vi "Cutlogfiles.vi"() -> ()   [LabVIEW 2018]
uses:
  <vilib>/Enthought/Python Integration Toolkit/api/Console Visibility.ctl
  Global Variables.vi
  <vilib>/Enthought/Python Integration Toolkit/Python Integration Toolkit.lvlib
panel:
  in  "Sample Rate":i32=100
  in  "New file":bool
  in  "selected path":path=path "C:/Labview Test Data/2018-08-13/Sensors/Log_Sensors_DAQ_0.tdms"
  out "XY Graph 2":cluster{dbl, "YScale.Maximum":dbl}[](graph)=[{3617058104.92992, "YScale.Maximum"=0.02}, {3617058117.2644606, "YScale.Maximum"=0.02}]
  out "XY Graph":cluster{dbl[], dbl[]}(graph)={[3617058104.92992, 3617058105.071405, 3617058105.204719, 3617058105.339352, 3617058105.4654217, 3617058105.5895977, 3617058105.723924, 3617058105.8577886, 3617058105.9931545, 3617058106.126216, 3617058106.2686815, 3617058106.402235, 3617058106.5402184, 3617058106.6768394, 3617058106.8146977, 3617058106.9502025, 3617058107.086078, 3617058107.2211895, 3617058107.3549776, 3617058107.4918585, 3617058107.627911, 3617058107.762443, 3617058107.901148, 3617058108.034609, 3617058108.171561, 3617058108.3105903, 3617058108.448009, 3617058108.586817, 3617058108.725321, 3617058108.86412, 3617058108.9984703, 3617058109.136935, 3617058109.275936, 3617058109.415624, 3617058109.5444145, 3617058109.6839633, 3617058109.8212304, 3617058109.959656, 3617058110.099505, 3617058110.2352777, 3617058110.37625, 3617058110.5166783, 3617058110.654278, 3617058110.792069, 3617058110.9294696, 3617058111.0667214, 3617058111.2080984, 3617058111.3436384, 3617058111.4812026, 3617058111.6171255, 3617058111.754656, 3617058111.8906007, 3617058112.028036, 3617058112.1654263, 3617058112.3010263, 3617058112.437075, 3617058112.5742207, 3617058112.7098174, 3617058112.847483, 3617058112.984029, 3617058113.11964, 3617058113.256136, 3617058113.395491, 3617058113.5323257, 3617058113.6705136, 3617058113.8095255, 3617058113.945854, 3617058114.0845695, 3617058114.2227335, 3617058114.360228, 3617058114.496631, 3617058114.634196, 3617058114.77004, 3617058114.90852, 3617058115.0450034, 3617058115.1819854, 3617058115.318167, 3617058115.4536457, 3617058115.591485, 3617058115.7283754, 3617058115.870709, 3617058116.009808, 3617058116.147975, 3617058116.2889624, 3617058116.4316134, 3617058116.575004, 3617058116.7180977, 3617058116.860796, 3617058117.000852, 3617058117.1353416, 3617058117.2644606], array[9200 elements]}
  out "Selected Channel":u32=2
  in  "stop":bool
  in  "Array":string[](array[string])=["Current_0", "Current_1", "Current_2", "Current_3", "Current_4", "Current_5", "Current_6", "Current_7"]
  in  "Cut":bool
  in  "Final Time":timestamp=timestamp(3617058117.2644606 s since 1904-01-01) format="%<%X\n%x>T"
  in  "Inital Time":timestamp=timestamp(3617058104.92992 s since 1904-01-01) format="%<%X\n%x>T"
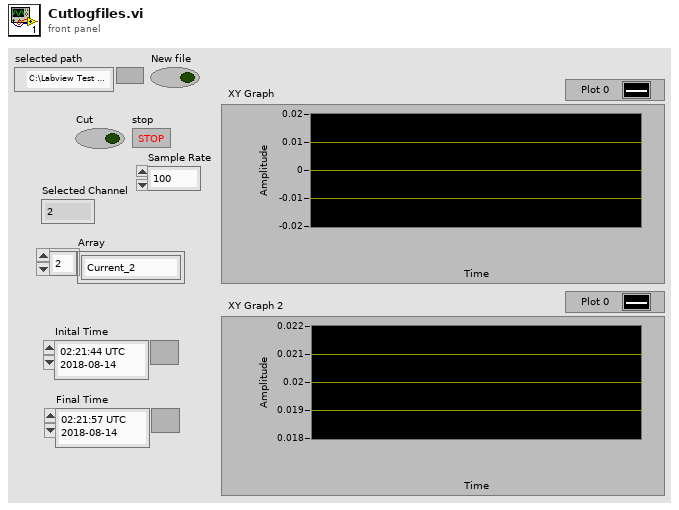
[diagram p1: front panel]
types:
  T1 = typedef "Python Integration Toolkit.lvlib/Console Visibility.ctl" = enum16{"Show Console", "Show Console While Running", "Hide Console"}
  T2 = enum16{"open", "open or create", "create or replace", "create", "open (read-only)"}
  T3 = typedef "Python Integration Toolkit.lvlib/Session ID.ctl" = u64
  T4 = typedef "Python Integration Toolkit.lvlib/Python Objects.ctl" = variant
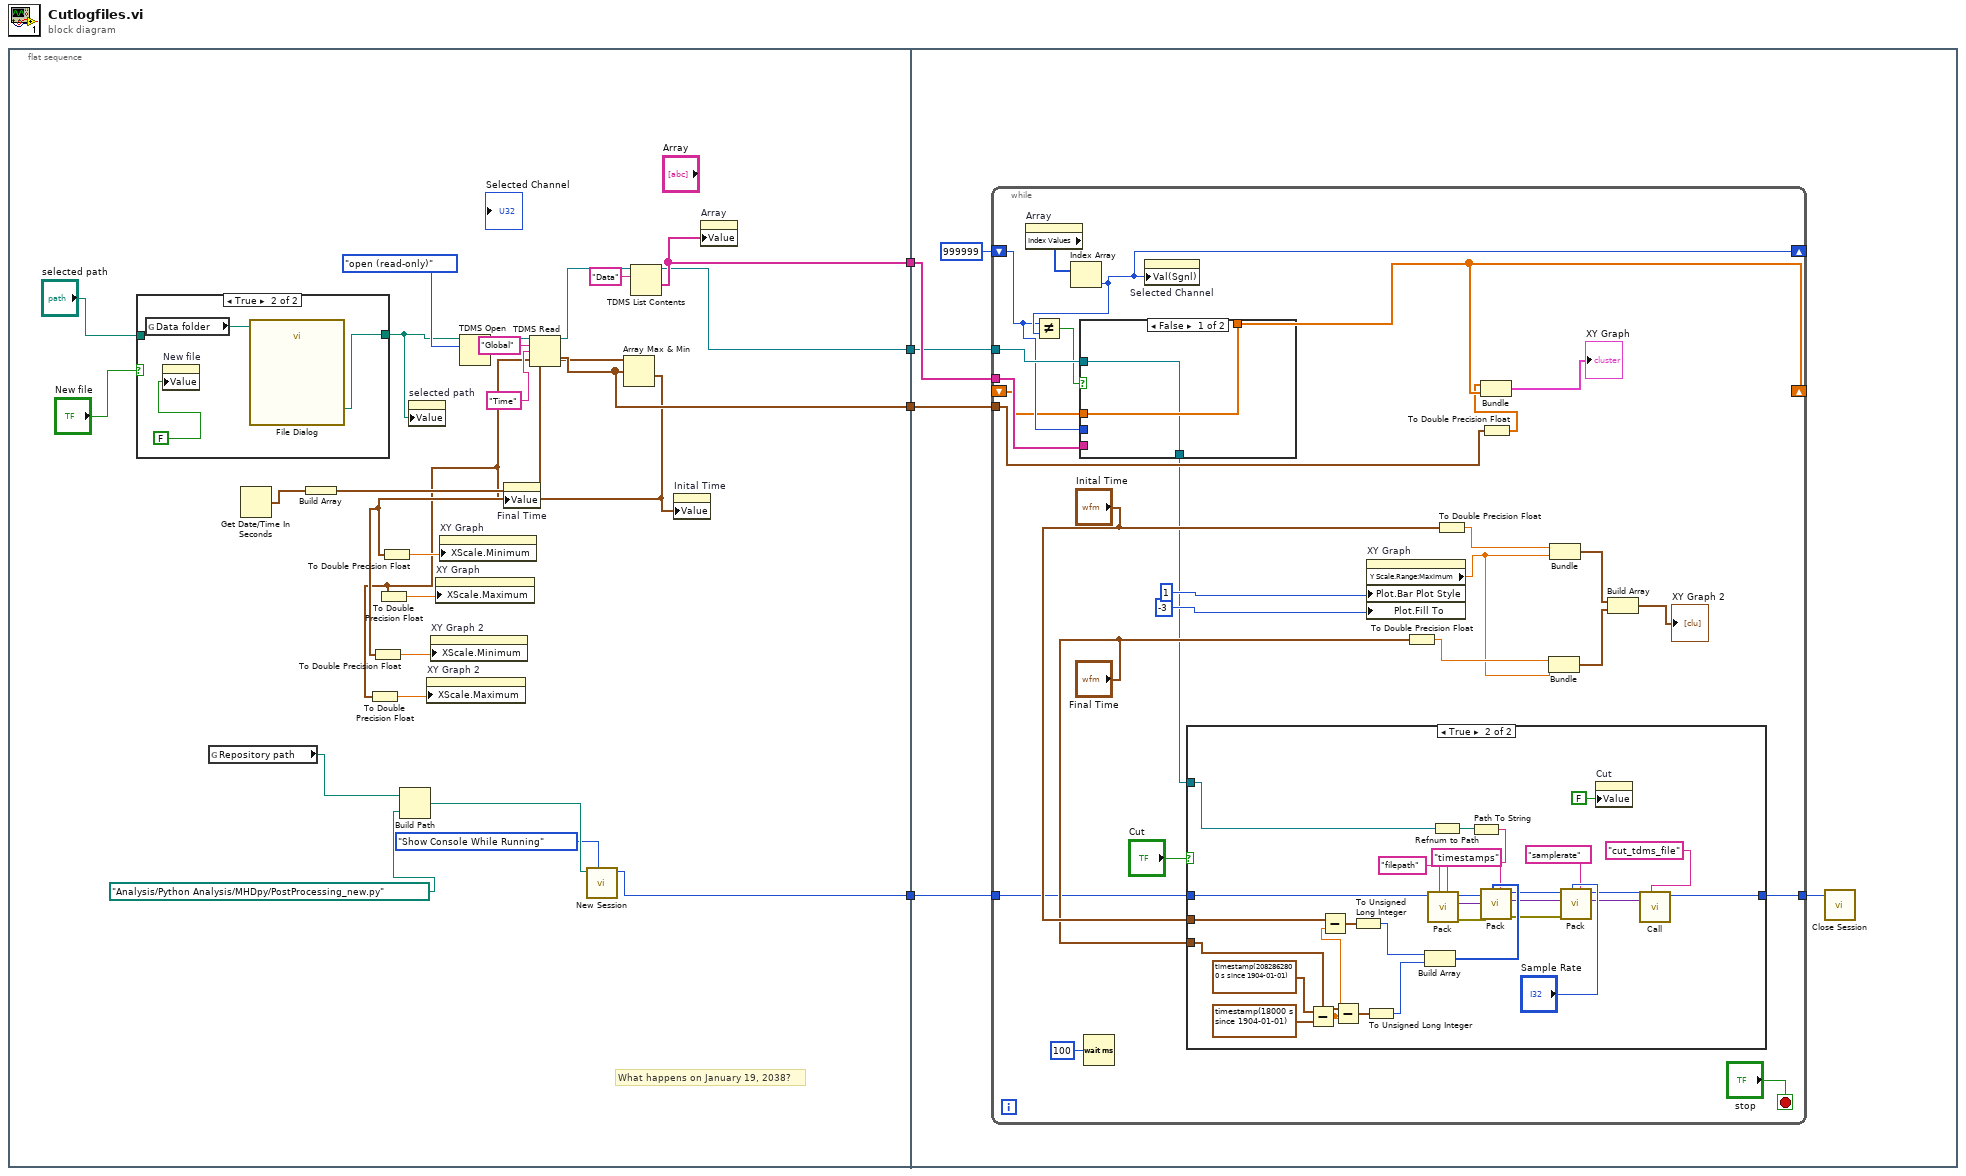
[diagram p0: block diagram]
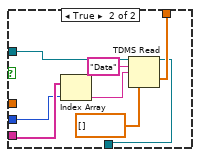
[diagram p4: hidden frame]
diagram:
  n1 = flat-sequence {
    tunnel: [w21] -> w4
    tunnel: [w19] -> w3
    tunnel: [w20] -> w2
    tunnel: [w10] -> w1
    tunnel: w4 -> [w39]
    tunnel: w3 -> [w38]
    tunnel: w2 -> [w37]
    tunnel: w1 -> [w35]
    frame #0 {
      # "What happens on January 19, 2038?"
      n2 = case shown="True" "New file" {
        tunnel: [w30 w32] -> w7
        tunnel: "selected path" -> [w30 _]
        frame False {
        }
        frame True {
          n3 = global read "Global Variables.vi" "Data folder"() -> (w33:path)
          n4 = property on="New file" class="Bool (strict)"("Value"=FALSE ("New file")) -> ()  [unwired: 2 in, 2 out]
          n5 = call "File Dialog"("start path"=w33) -> ("selected path"=w32:path)  [unwired: 11 in, 3 out]
        }
      }
      n6 = global read "Global Variables.vi" "Repository path"() -> (w12:path)
      n7 = Get Date/Time In Seconds() -> (seconds since 1Jan1904=w25:timestamp)
      n8 = Build Array(w25) -> (w24:timestamp[])
      n9 = Build Path(base path=w12, name or relative path=path "Analysis/Python Analysis/MHDpy/PostProcessing_new.py" ("Repository path")) -> (appended path=w9:path)
      n10 = property on="selected path" class="Path"("Value"=w7) -> ()  [unwired: 2 in, 2 out]
      n11 = TDMS Open(10:T2."open (read-only)" ("operation (0:open)"), 11:w7) -> (3:w28:refnum<k34>)  [unwired: 5 in, 1 out]
      n12 = TDMS Read(0:w28, 5:"Global" ("group name in"), 7:"Time" ("group name in"), 12:w24) -> (4:w23:refnum<k34>, 10:w19:timestamp[])  [unwired: 4 in, 4 out]
      n13 = call <vilib>:"New Session.vi"("Console Visibility"=Console_Visibility."Show Console While Running", "Path to Python Module (.py File)"=w9) -> ("Session ID out"=w10:T3)  [unwired: 8 in, 1 out]
      n14 = Array Max & Min(array=w19) -> (max value=w13:timestamp, min value=w14:timestamp)  [unwired: 2 out]
      n15 = To Double Precision Float(number=w13) -> (double precision float=w16:dbl)
      n16 = To Double Precision Float(number=w14) -> (double precision float=w15:dbl)
      n17 = To Double Precision Float(number=w13) -> (double precision float=w17:dbl)
      n18 = To Double Precision Float(number=w14) -> (double precision float=w18:dbl)
      n19 = property on="XY Graph 2" class="XYGraph (strict)"("XScale.Maximum"=w16) -> ()  [unwired: 2 in, 2 out]
      n20 = property on="XY Graph 2" class="XYGraph (strict)"("XScale.Minimum"=w15) -> ()  [unwired: 2 in, 2 out]
      n21 = property on="XY Graph" class="XYGraph (strict)"("XScale.Maximum"=w17) -> ()  [unwired: 2 in, 2 out]
      n22 = property on="XY Graph" class="XYGraph (strict)"("XScale.Minimum"=w18) -> ()  [unwired: 2 in, 2 out]
      n23 = property on="Final Time" class="AbsTime (strict)"("Value"=w13) -> ()  [unwired: 2 in, 2 out]
      n24 = TDMS List Contents(6:"Data" ("group name"), 7:w23) -> (1:w21:string[], 3:w20:refnum<k34>)  [unwired: 1 in, 2 out]
      n25 = property on="Inital Time" class="AbsTime (strict)"("Value"=w14) -> ()  [unwired: 2 in, 2 out]
      n26 = property on="Array" class="Arr (strict)"("Value"=w21) -> ()  [unwired: 2 in, 2 out]
    }
    frame #1 {
      n27 = while {
        tunnel: w38 -> [w57]
        tunnel: w37 -> [w62]
        tunnel: w39 -> [w63]
        shift-right: [w56] -> _
        shift-left: _ -> [w58]
        shift-right: [w61] -> _
        shift-left: u32 999999 -> [w59]
        tunnel: w35 -> [w43]
        tunnel: [w41] -> w34
        stop <- "stop" stop-if-true
        n28 = property on="Array" class="Arr (strict)"() -> ("Index Values"=w64:u32[])  [unwired: 2 in, 2 out]
        n29 = Index Array(array=w64) -> (element=w61:u32)  [unwired: 1 in]
        n30 = Not Equal?(x=w59, y=w61) -> (x != y?=w60:bool)
        n31 = case shown="False" w60 {
          tunnel: w63 -> [_ w106]
          tunnel: w62 -> [w97 w105]
          tunnel: [w98 w104] -> w56
          tunnel: w59 -> [_ w101]
          tunnel: w58 -> [w98 _]
          tunnel: [w97 w99] -> w42
          frame False {
          }
          frame True {
            n32 = Index Array(array=w106, index=w101) -> (element=w102:string)
            n33 = TDMS Read(0:w105, 5:"Data" ("group name in"), 7:w102, 12:dbl[] []) -> (4:w99:refnum<k34>, 10:w104:dbl[])  [unwired: 4 in, 4 out]
          }
        }
        n34 = Wait (ms)(milliseconds to wait=u32 100) -> ()  [unwired: 1 out]
        n35 = property on="Selected Channel" class="DigNum (strict)"("Val(Sgnl)"=w61) -> ()  [unwired: 2 in, 2 out]
        n36 = case shown="True" "Cut" {
          tunnel: "Inital Time" -> [_ w71]
          tunnel: "Final Time" -> [_ w70]
          tunnel: w43 -> [w67 w94]
          tunnel: w42 -> [_ w96]
          tunnel: [w67 w93] -> w41
          frame False {
          }
          frame True {
            n37 = Subtract(x=timestamp(2082862800 s since 1904-01-01) ("current time"), y=timestamp(18000 s since 1904-01-01) ("current time")) -> (x-y=w72:dbl)
            n38 = Subtract(x=w71, y=w72) -> (x-y=w73:timestamp)
            n39 = Subtract(x=w70, y=w72) -> (x-y=w76:timestamp)
            n40 = To Unsigned Long Integer(number=w73) -> (unsigned 32bit integer=w69:u32)
            n41 = To Unsigned Long Integer(number=w76) -> (unsigned 32bit integer=w68:u32)
            n42 = Build Array(w69, w68) -> (w88:u32[])
            n43 = Refnum to Path(1:w96) -> (0:w95:path)
            n44 = Path To String(path=w95) -> (string=w87:string)
            n45 = call <vilib>:"Pack.vi"("Keyword Name"="filepath", "Argument"=w87, "Session ID"=w94) -> ("error out"=w91:errorcluster, "Python Object References Out"=w90:T4, "Session ID out"=w89:T3)  [unwired: 6 in]
            n46 = call <vilib>:"Pack.vi"("Keyword Name"="timestamps", "Argument"=w88, "error in (no error)"=w91, "Python Object References In"=w90, "Session ID"=w89) -> ("error out"=w83:errorcluster, "Python Object References Out"=w82:T4, "Session ID out"=w81:T3)  [unwired: 4 in]
            n47 = call <vilib>:"Pack.vi"("Keyword Name"="samplerate", "Argument"="Sample Rate", "error in (no error)"=w83, "Python Object References In"=w82, "Session ID"=w81) -> ("Python Object References Out"=w77:T4, "Session ID out"=w78:T3)  [unwired: 4 in, 1 out]
            n48 = property on="Cut" class="Bool (strict)"("Value"=FALSE ("Cut")) -> ()  [unwired: 2 in, 2 out]
            n49 = call <vilib>:"Call.vi"("Function or Method Name"="cut_tdms_file" ("Keyword Name"), "Python Object References In"=w77, "Session ID"=w78) -> ("Session ID out"=w93:T3)  [unwired: 6 in, 2 out]
          }
        }
        n50 = property on="XY Graph" class="XYGraph (strict)"("Plot.Bar Plot Style"=u8 1, "Plot.Fill To"=i16 -3) -> ("Y Scale.Range:Maximum"=w46:dbl)  [unwired: 2 in, 2 out]
        n51 = To Double Precision Float(number="Final Time") -> (double precision float=w51:dbl)
        n52 = To Double Precision Float(number="Inital Time") -> (double precision float=w52:dbl)
        n53 = To Double Precision Float(number=w57) -> (double precision float=w55:dbl[])
        n54 = Bundle(w55, w56) -> (→"XY Graph":cluster{dbl[], dbl[]})  [unwired: 1 in]
        n55 = Bundle(w51, "YScale.Maximum"=w46) -> (w48:cluster{dbl, "YScale.Maximum":dbl})  [unwired: 1 in]
        n56 = Bundle(w52, "YScale.Maximum"=w46) -> (w49:cluster{dbl, "YScale.Maximum":dbl})  [unwired: 1 in]
        n57 = Build Array(w49, w48) -> (→"XY Graph 2":cluster{dbl, "YScale.Maximum":dbl}[])
      }
      n58 = call <vilib>:"Close Session.vi"("Session ID"=w34) -> ()  [unwired: 10 in, 1 out]
    }
  }
